vi "map (un)bundle to subVI.vi"(8 "error in (no error)":errorcluster, 10 "Terms[]":refnum<vi>[](array[refnum]), 11 "SubVI in":refnum<vi>) -> (0 "error out":errorcluster)   [LabVIEW 2013]
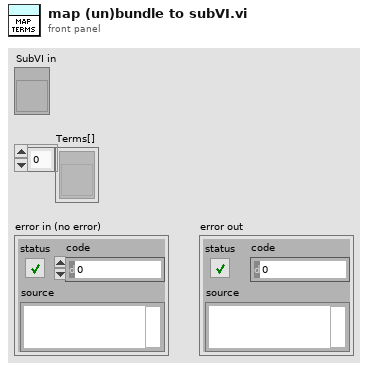
[diagram p1: front panel]
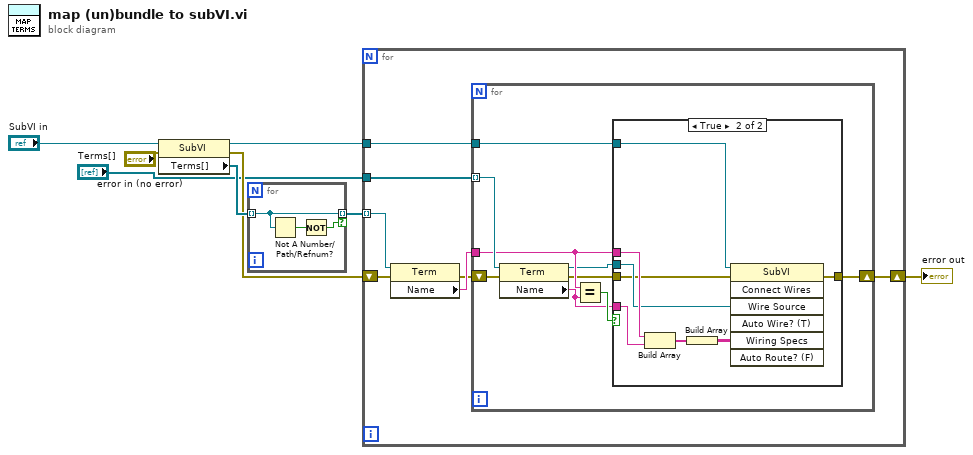
[diagram p0: block diagram]
diagram:
  n1 = property class="SubVI"(reference="SubVI in", error in="error in (no error)") -> (reference out=w6:refnum<vi>, error out=w4:errorcluster, "Terms[]"=w7:refnum<vi>[])
  n2 = for {
    tunnel: w7 -> [w11] mode=indexing
    tunnel: [w11] -> w8 mode=indexing if=w9
    n3 = Not A Number/Path/Refnum?(number/path/refnum=w11) -> (NaN/Path/Refnum?=w10:bool)
    n4 = Not(x=w10) -> (.not. x?=w9:bool)
  }
  n5 = for {
    tunnel: "Terms[]" -> [w18]
    tunnel: w6 -> [w16]
    shift-right: [w13] -> w5
    shift-left: w4 -> [w15]
    tunnel: w8 -> [w12] mode=indexing
    n6 = property class="Term"(reference=w12, error in=w15) -> (error out=w14:errorcluster, "Name"=w17:string)  [unwired: 1 out]
    n7 = for {
      tunnel: w18 -> [w27] mode=indexing
      tunnel: w17 -> [w23]
      tunnel: w16 -> [w26]
      shift-right: [w19] -> w13
      shift-left: w14 -> [w21]
      n8 = property class="Term"(reference=w27, error in=w21) -> (reference out=w22:refnum<vi>, error out=w20:errorcluster, "Name"=w24:string)
      n9 = Equal?(x=w23, y=w24) -> (x = y?=w25:bool)
      n10 = case shown="True" w25 {
        tunnel: w26 -> [_ w36]
        tunnel: w24 -> [_ w35]
        tunnel: w23 -> [_ w34]
        tunnel: w22 -> [_ w31]
        tunnel: w20 -> [w28 w30]
        tunnel: [w28 w29] -> w19
        frame False {
        }
        frame True {
          n11 = Build Array(w34, w35) -> (w33:string[])
          n12 = Build Array(w33) -> (w32:string[][])
          n13 = invoke class="SubVI" method="Connect Wires"(reference=w36, error in=w30, "Wire Source"=w31, "Wiring Specs"=w32) -> (error out=w29:errorcluster)  [unwired: 3 in, 6 out]
        }
      }
    }
  }
  "error out" <- w5
